vi "TCP Receive Server.vi"() -> ()   [LabVIEW 2010]
doc: "Sends a specified waveform through a TCP port. The VI first listens for a connection and, once established, sends the number of bytes to be sent followed by the data. After the data is sent, the VI waits for an 'all received' signal from the client and then breaks the connection.\n\n<B>Note:</B> Requires the Data Client.vi located in the same library as this VI."
uses:
  3.0 Flow Control/3.0 List of Loops.ctl
  3.0-Global.vi
panel:
  in  "Port":u16=53483 min=1025 step=1
  # "Instructions:\n1. Open the Data Client.vi\n2. Run This VI first.\n3. Run the Data Client.vi Second.\n4. Adjust the # of Points Function, and Noise Level controls.\n5. Observe the Chart on the Data Client.vi.\n6. Stop This VI. The Data Client.vi will time out and stop."
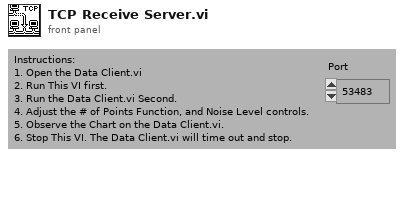
[diagram p1: front panel]
types:
  T1 = typedef "3.0 List of Loops.ctl" = enum16{"3.0 State Update", "3.0 GUI", "3.1 Act", "3.1 4.7.1 Act UDP", "3.1 Joystick", "3.2 Where", "3.2 4.7.2 Where UDP", "3.3 What", "3.3 4.7.3 What UDP", "3.4 How", "3.4 4.7.4 How UDP", "3.5 Limbic", "3.8 TCP", "3.6 Cerebellum", "3.8 TCP Act"}
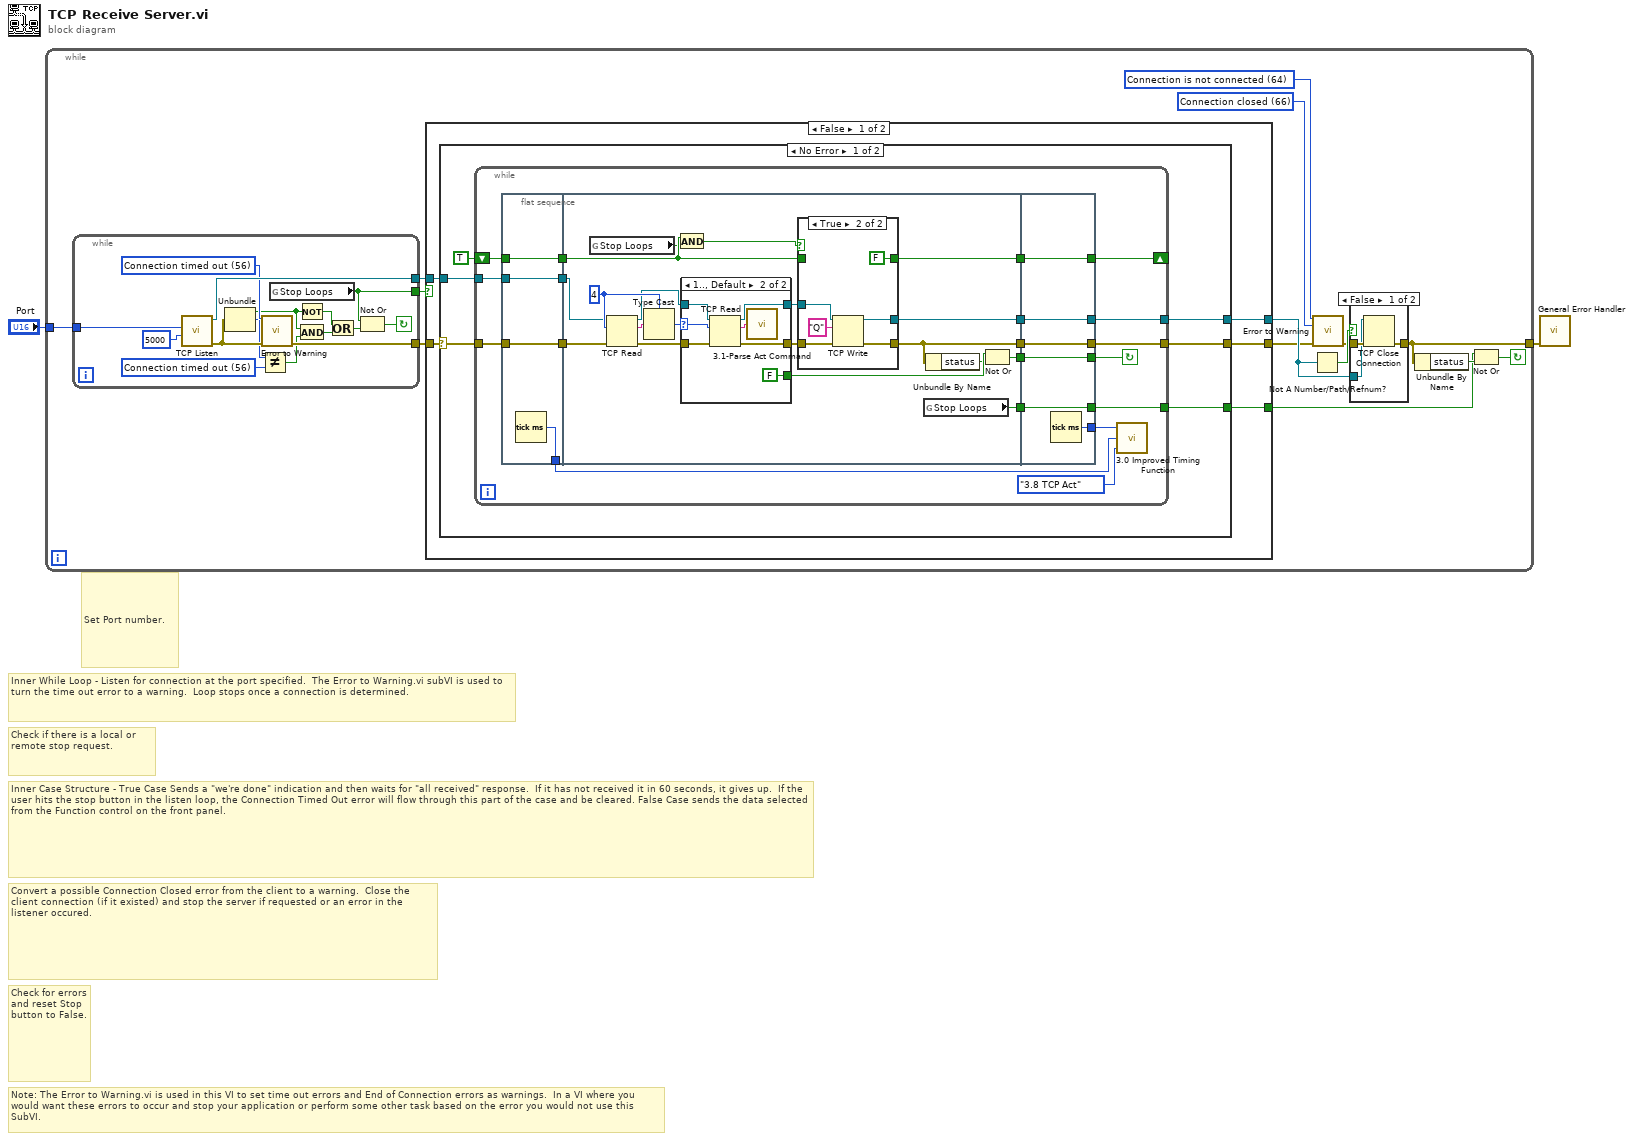
[diagram p0: block diagram]
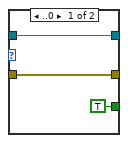
[diagram p3: hidden frame]
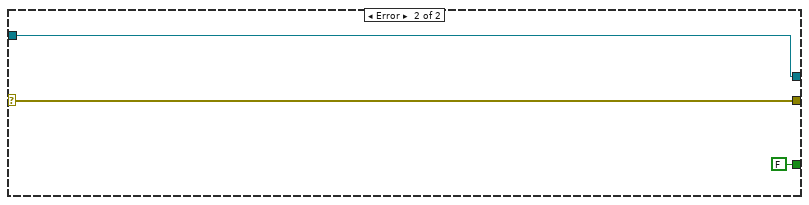
[diagram p4: hidden frame]
diagram:
  # "Check for errors\nand reset Stop \nbutton to False."
  # "Inner Case Structure - True Case Sends a \"we're done\" indication and then waits for \"all received\" response.  If it has not received it in 60 seconds, it gives up.  If the user hits the stop button in the listen loop, the Connection Timed Out error will flow through this part of the case and be cleared. False Case sends the data selected from the Function control on the front panel."
  # "Check if there is a local or remote stop request."
  # "Set Port number."
  # "Inner While Loop - Listen for connection at the port specified.  The Error to Warning.vi subVI is used to turn the time out error to a warning.  Loop stops once a connection is determined."
  # "Note: The Error to Warning.vi is used in this VI to set time out errors and End of Connection errors as warnings.  In a VI where you would want these errors to occur and stop your application or perform some other task based on the error you would not use this SubVI."
  # "Convert a possible Connection Closed error from the client to a warning.  Close the client connection (if it existed) and stop the server if requested or an error in the listener occured."
  n1 = while {
    tunnel: [w9] -> w1
    tunnel: "Port" -> [w15]
    stop <- w16 continue-if-true
    w5 = 66 items=["No Error", "Argument Error", "Memory Full", "Out of Zone", "End of File", "File Already Open", "Generic File IO Error", "File Not Found", "File Permission Error", "Disk Full", "Duplicate Path", "Too Many Files Open", "Not Enabled", "Resource File Not Found", "Cannot Add Resource", "Resource Not Found", "Image Not Found", "Image Memory Error", "Pen Does Not Exist", "Config Bad Type", "Config Token Not Found", "Config Parse Error", "Config Memory Error", "Bad External Code Format", "Bad External Code Offset", "External Code Not Present", "Null Window", "Destroy Window Mixup", "Null Menu", "Print Aborted", "Bad Print Record", "Print Driver Error", "Windows Error During Print", "Memory Error During Print", "Print Dialog Error", "Generic Print Error", "Invalid Device Refnum", "Device Not Found", "Device Parameter Error", "Device Unit Error", "Can't Open Device", "Device Call Aborted", "Generic Error", "Cancelled By User", "Object ID Too Low", "Object ID Too High", "Object Not In Heap", "Unknown Heap", "Bad DefProc ID", "DefProc Not In Table", "Message Out Of Range", "Null Method", "Unknown Message", "Manager Call Not Supported", "Bad address", "Connection In progress", "Connection timed out", "Connection is already in progress", "Network attribute not supported", "Network error", "Address in use", "System out of memory", "Connection aborted", "Connection refused", "Connection is not connected", "Connection is already connected", "Connection closed", "Initialize error (interapplication manager)", "Bad occurrence", "Wait on unbound occurrence handler", "Occurrence queue overflow", "Bad path", "Semaphore not signaled", "Unrecognized type (interapplication manager)"] ("2nd Error to Convert")
    w6 = 64 items=["No Error", "Argument Error", "Memory Full", "Out of Zone", "End of File", "File Already Open", "Generic File IO Error", "File Not Found", "File Permission Error", "Disk Full", "Duplicate Path", "Too Many Files Open", "Not Enabled", "Resource File Not Found", "Cannot Add Resource", "Resource Not Found", "Image Not Found", "Image Memory Error", "Pen Does Not Exist", "Config Bad Type", "Config Token Not Found", "Config Parse Error", "Config Memory Error", "Bad External Code Format", "Bad External Code Offset", "External Code Not Present", "Null Window", "Destroy Window Mixup", "Null Menu", "Print Aborted", "Bad Print Record", "Print Driver Error", "Windows Error During Print", "Memory Error During Print", "Print Dialog Error", "Generic Print Error", "Invalid Device Refnum", "Device Not Found", "Device Parameter Error", "Device Unit Error", "Can't Open Device", "Device Call Aborted", "Generic Error", "Cancelled By User", "Object ID Too Low", "Object ID Too High", "Object Not In Heap", "Unknown Heap", "Bad DefProc ID", "DefProc Not In Table", "Message Out Of Range", "Null Method", "Unknown Message", "Manager Call Not Supported", "Bad address", "Connection In progress", "Connection timed out", "Connection is already in progress", "Network attribute not supported", "Network error", "Address in use", "System out of memory", "Connection aborted", "Connection refused", "Connection is not connected", "Connection is already connected", "Connection closed", "Initialize error (interapplication manager)", "Bad occurrence", "Wait on unbound occurrence handler", "Occurrence queue overflow", "Bad path", "Semaphore not signaled", "Unrecognized type (interapplication manager)"] ("1st Error to Convert")
    n2 = while {
      tunnel: [w17] -> w12
      tunnel: [w26] -> w13
      tunnel: [w30] -> w14
      tunnel: w15 -> [w31]
      stop <- w28 continue-if-true
      w24 = 56 items=["No Error", "Argument Error", "Memory Full", "Out of Zone", "End of File", "File Already Open", "Generic File IO Error", "File Not Found", "File Permission Error", "Disk Full", "Duplicate Path", "Too Many Files Open", "Not Enabled", "Resource File Not Found", "Cannot Add Resource", "Resource Not Found", "Image Not Found", "Image Memory Error", "Pen Does Not Exist", "Config Bad Type", "Config Token Not Found", "Config Parse Error", "Config Memory Error", "Bad External Code Format", "Bad External Code Offset", "External Code Not Present", "Null Window", "Destroy Window Mixup", "Null Menu", "Print Aborted", "Bad Print Record", "Print Driver Error", "Windows Error During Print", "Memory Error During Print", "Print Dialog Error", "Generic Print Error", "Invalid Device Refnum", "Device Not Found", "Device Parameter Error", "Device Unit Error", "Can't Open Device", "Device Call Aborted", "Generic Error", "Cancelled By User", "Object ID Too Low", "Object ID Too High", "Object Not In Heap", "Unknown Heap", "Bad DefProc ID", "DefProc Not In Table", "Message Out Of Range", "Null Method", "Unknown Message", "Manager Call Not Supported", "Bad address", "Connection In progress", "Connection timed out", "Connection is already in progress", "Network attribute not supported", "Network error", "Address in use", "System out of memory", "Connection aborted", "Connection refused", "Connection is not connected", "Connection is already connected", "Connection closed", "Initialize error (interapplication manager)", "Bad occurrence", "Wait on unbound occurrence handler", "Occurrence queue overflow", "Bad path", "Semaphore not signaled", "Unrecognized type (interapplication manager)"] ("1st Error to Convert")
      w25 = 56 items=["No Error", "Argument Error", "Memory Full", "Out of Zone", "End of File", "File Already Open", "Generic File IO Error", "File Not Found", "File Permission Error", "Disk Full", "Duplicate Path", "Too Many Files Open", "Not Enabled", "Resource File Not Found", "Cannot Add Resource", "Resource Not Found", "Image Not Found", "Image Memory Error", "Pen Does Not Exist", "Config Bad Type", "Config Token Not Found", "Config Parse Error", "Config Memory Error", "Bad External Code Format", "Bad External Code Offset", "External Code Not Present", "Null Window", "Destroy Window Mixup", "Null Menu", "Print Aborted", "Bad Print Record", "Print Driver Error", "Windows Error During Print", "Memory Error During Print", "Print Dialog Error", "Generic Print Error", "Invalid Device Refnum", "Device Not Found", "Device Parameter Error", "Device Unit Error", "Can't Open Device", "Device Call Aborted", "Generic Error", "Cancelled By User", "Object ID Too Low", "Object ID Too High", "Object Not In Heap", "Unknown Heap", "Bad DefProc ID", "DefProc Not In Table", "Message Out Of Range", "Null Method", "Unknown Message", "Manager Call Not Supported", "Bad address", "Connection In progress", "Connection timed out", "Connection is already in progress", "Network attribute not supported", "Network error", "Address in use", "System out of memory", "Connection aborted", "Connection refused", "Connection is not connected", "Connection is already connected", "Connection closed", "Initialize error (interapplication manager)", "Bad occurrence", "Wait on unbound occurrence handler", "Occurrence queue overflow", "Bad path", "Semaphore not signaled", "Unrecognized type (interapplication manager)"] ("1st Error to Convert")
      n3 = call <vilib>:"TCP Listen.vi"("timeout ms (wait forever: -1)"=5000, "port"=w31) -> ("error out"=w27:errorcluster, "connection ID"=w30:refnum<k5>)  [unwired: 6 in, 2 out]
      n4 = Unbundle(w27) -> ("status"=w22:bool, "code"=w23:i32)  [unwired: 1 out]
      n5 = Not Equal?(x=w23, y=w24) -> (x != y?=w21:bool)
      n6 = call <vilib>:"Error to Warning.vi"("1st Error to Convert"=w25, "error in"=w27) -> ("warning out"=w26:errorcluster)  [unwired: 13 in]
      n7 = global read "3.0-Global.vi" "Stop Loops"() -> (w17:bool)
      n8 = Not(x=w22) -> (.not. x?=w20:bool)
      n9 = And(x=w22, y=w21) -> (x .and. y?=w19:bool)
      n10 = Or(x=w20, y=w19) -> (x .or. y?=w18:bool)
      n11 = Not Or(1:w18, 2:w17) -> (0:w28:bool)
    }
    n12 = case shown="False" w12 {
      selector: w12 -> [_ w113]
      tunnel: [w36 w114] -> w4
      tunnel: w14 -> [w35 w115]
      tunnel: w13 -> [w32 w114]
      tunnel: [w34 w115] -> w11
      tunnel: [w33 w113] -> w7
      frame False {
        n13 = case shown="No Error" w32 {
          selector: w32 -> [w41 w110]
          tunnel: [w39 w110] -> w36
          tunnel: w35 -> [w42 w112]
          tunnel: [w40 w112] -> w34
          tunnel: [w38 FALSE] -> w33
          frame No Error {
            n14 = while {
              shift-left: TRUE -> [w58]
              shift-right: [w60] -> _
              tunnel: [w59] -> w40
              tunnel: [w57] -> w39
              tunnel: w42 -> [w56]
              tunnel: w41 -> [w55]
              tunnel: [w54] -> w38
              stop <- w61 continue-if-true
              n15 = flat-sequence {
                tunnel: w55 -> [w63]
                tunnel: w56 -> [w64]
                tunnel: w58 -> [w65]
                tunnel: [w65] -> w48
                tunnel: [w64] -> w47
                tunnel: [w63] -> w46
                tunnel: [w62] -> w44
                tunnel: [w83] -> w53
                tunnel: [w79] -> w52
                tunnel: [w74] -> w51
                tunnel: [w71] -> w50
                tunnel: [w66] -> w49
                tunnel: w48 -> [w72]
                tunnel: w47 -> [w69]
                tunnel: w46 -> [w68]
                tunnel: [w105] -> w54
                tunnel: [w106] -> w57
                tunnel: [w107] -> w59
                tunnel: [w108] -> w60
                tunnel: [w109] -> w61
                tunnel: w53 -> [w109]
                tunnel: w52 -> [w108]
                tunnel: w51 -> [w107]
                tunnel: w50 -> [w106]
                tunnel: w49 -> [w105]
                tunnel: [w104] -> w45
                frame #0 {
                  n16 = Tick Count (ms)() -> (millisecond timer value=w62:u32)
                }
                frame #1 {
                  w82 = 4
                  n17 = global read "3.0-Global.vi" "Stop Loops"() -> (w67:bool)
                  n18 = TCP Read(connection ID=w69, bytes to read=w82, error in (no error)=w68) -> (connection ID out=w75:refnum<k5>, data out=w84:string, error out=w76:errorcluster)  [unwired: 2 out]
                  n19 = Type Cast(type=w82, x=w84) -> (*(type *) &x=w81:i32)
                  n20 = And(x=w72, y=w67) -> (x .and. y?=w80:bool)
                  n21 = case shown="1.., Default" w81 {
                    selector: w81 -> [_ w100]
                    tunnel: w76 -> [w94 w103]
                    tunnel: w75 -> [w96 w102]
                    tunnel: [w96 w101] -> w73
                    tunnel: [TRUE FALSE] -> w77
                    tunnel: [w94 w98] -> w78
                    frame ..0 {
                    }
                    frame 1.., Default {
                      n22 = TCP Read(connection ID=w102, bytes to read=w100, error in (no error)=w103) -> (connection ID out=w101:refnum<k5>, data out=w97:string, error out=w98:errorcluster)  [unwired: 2 out]
                      n23 = call "3.1-Parse Act Command.vi"("data out"=w97) -> ()
                    }
                  }
                  n24 = case shown="True" w80 {
                    tunnel: w72 -> [w86 _]
                    tunnel: [w86 FALSE] -> w79
                    tunnel: w73 -> [w85 w93]
                    tunnel: w78 -> [w87 w90]
                    tunnel: [w87 w89] -> w71
                    tunnel: [w85 w88] -> w74
                    frame False {
                    }
                    frame True {
                      n25 = TCP Write(connection ID=w93, data in="Q", error in (no error)=w90) -> (connection ID out=w88:refnum<k5>, error out=w89:errorcluster)  [unwired: 2 out]
                    }
                  }
                  n26 = global read "3.0-Global.vi" "Stop Loops"() -> (w66:bool)
                  n27 = Unbundle By Name(w71) -> ("status"=w70:bool)
                  n28 = Not Or(1:w70, 2:w77) -> (0:w83:bool)
                }
                frame #2 {
                  n29 = Tick Count (ms)() -> (millisecond timer value=w104:u32)
                }
              }
              n30 = call "3.0 Improved Timing Function.vi"("Loop"=3.0_List_of_Loops."3.8 TCP Act", "Start"=w44, "End"=w45) -> ()  [unwired: 1 in]
            }
          }
          frame Error {
          }
        }
      }
      frame True {
      }
    }
    n31 = Not A Number/Path/Refnum?(number/path/refnum=w11) -> (NaN/Path/Refnum?=w10:bool)
    n32 = call <vilib>:"Error to Warning.vi"("1st Error to Convert"=w6, "2nd Error to Convert"=w5, "error in"=w4) -> ("warning out"=w3:errorcluster)  [unwired: 12 in]
    n33 = case shown="False" w10 {
      tunnel: w3 -> [w118 w119]
      tunnel: w11 -> [w117 _]
      tunnel: [w116 w119] -> w9
      frame False {
        n34 = TCP Close Connection(connection ID=w117, error in (no error)=w118) -> (error out=w116:errorcluster)  [unwired: 1 in, 1 out]
      }
      frame True {
      }
    }
    n35 = Unbundle By Name(w9) -> ("status"=w8:bool)
    n36 = Not Or(1:w8, 2:w7) -> (0:w16:bool)
  }
  n37 = call <vilib>:"General Error Handler.vi"("error in (no error)"=w1) -> ()  [unwired: 10 in, 5 out]
